vi "SetRange.vi"(9 "Unit":string(combo)="POW", 10 "AUTO":bool, 11 "VISA in":refnum<visa-resource-name>="USB0::0x1313::0x8070::P0000118::INSTR") -> (0 "AUTO?":bool, 1 "RANG_Val":dbl, 2 "RANG_lbl":string, 4 "GetIndex":i16)   [LabVIEW 2015]
panel:
  out "Rng":string
  in  "Range":i16=1 min=1 max=4 step=1
  in  "stop":bool
  # "Set Measurement Range"
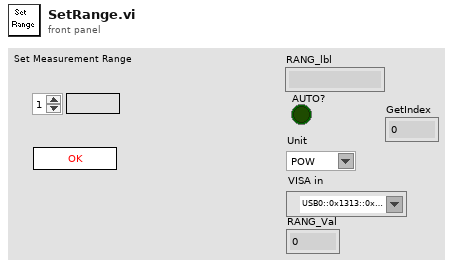
[diagram p1: front panel]
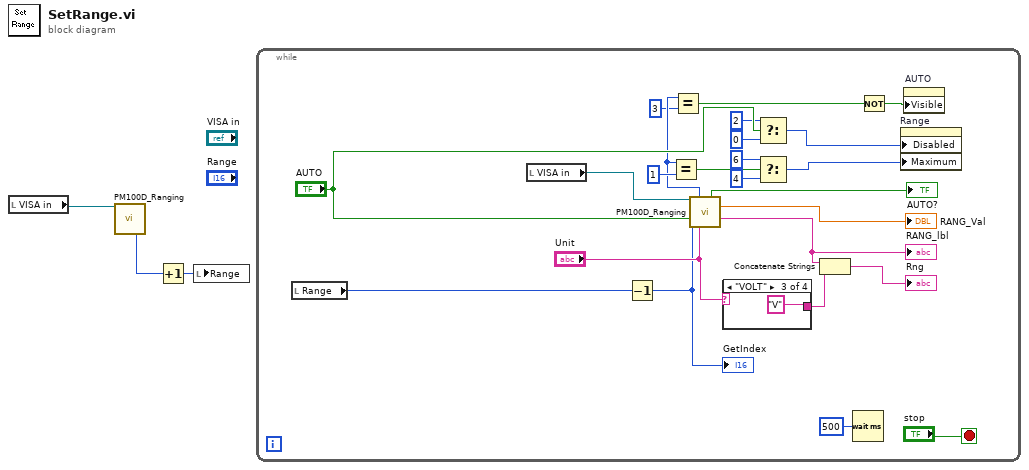
[diagram p0: block diagram]
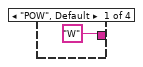
[diagram p2: hidden frame]
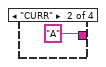
[diagram p3: hidden frame]
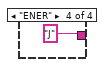
[diagram p4: hidden frame]
diagram:
  n1 = local read "VISA in"() -> (w1:refnum<visa-resource-name>)
  n2 = call "PM100D_Ranging.vi"("VISA in"=w1) -> ("IndexOut"=w2:i32)  [unwired: 7 in, 7 out]
  n3 = Increment(x=w2) -> (x+1=w3:i32)
  n4 = local write "Range"(w3) -> ()
  n5 = while {
    stop <- "stop" stop-if-true
    n6 = local read "Range"() -> (w5:i16)
    n7 = local read "VISA in"() -> (w4:refnum<visa-resource-name>)
    n8 = Decrement(x=w5) -> (x-1=w12:i16)
    "GetIndex" <- w12
    n9 = call "PM100D_Ranging.vi"("VISA in"=w4, "Index"=w12, "AUTO"="AUTO", "Unit"="Unit") -> ("SensType"=w11:i32, "AUTO?"=→"AUTO?":bool, "RANG_Val"=→"RANG_Val":dbl, "RANG_lbl"=w21:string)  [unwired: 4 in, 4 out]
    "RANG_lbl" <- w21
    n10 = Equal?(x=w11, y=1) -> (x = y?=w16:bool)
    n11 = Equal?(x=w11, y=3) -> (x = y?=w6:bool)
    n12 = case shown="\"VOLT\"" "Unit" {
      tunnel: ["W" "A" "V" "J"] -> w20
      frame "POW", Default {
      }
      frame "CURR" {
      }
      frame "VOLT" {
      }
      frame "ENER" {
      }
    }
    n13 = Select(t=2, s="AUTO", f=0) -> (s? t:f=w18:i32)
    n14 = Select(t=6, s=w16, f=4) -> (s? t:f=w17:i32)
    n15 = Concatenate Strings(w21, w20) -> (→"Rng":string)
    n16 = Wait (ms)(milliseconds to wait=u32 500) -> ()  [unwired: 1 out]
    n17 = Not(x=w6) -> (.not. x?=w7:bool)
    n18 = property on="Range" class="DigNum (strict)"("Disabled"=w18, "Maximum"=w17) -> ()  [unwired: 2 in, 2 out]
    n19 = property on="AUTO" class="Bool (strict)"("Visible"=w7) -> ()  [unwired: 2 in, 2 out]
  }
